vi "CoordLoadTemp.vi"(11 "appended path":path) -> (3 "CoordTempOut":T1[](array[typedef]))   [LabVIEW 2015]
uses:
  <vilib>/vision/Image Controls.llb/IMAQ Image.ctl
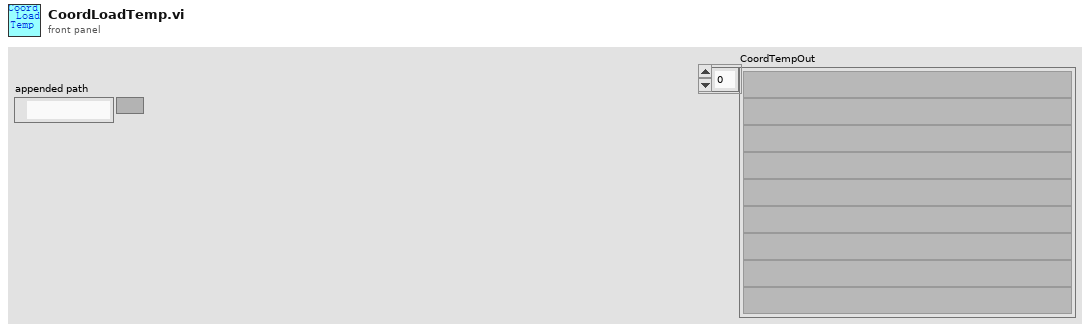
[diagram p1: front panel]
types:
  T1 = typedef "IMAQ Image.ctl" = refnum<image>
  T2 = typedef "Image Type" = u32
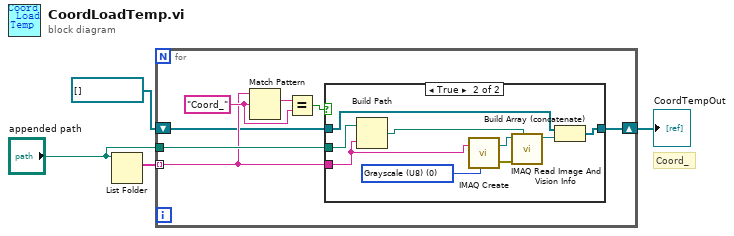
[diagram p0: block diagram]
diagram:
  # "Coord_"
  n1 = List Folder(path="appended path") -> (filenames=w4:string[])  [unwired: 3 in, 3 out]
  n2 = for {
    tunnel: w4 -> [w8] mode=indexing
    tunnel: "appended path" -> [w9]
    shift-right: [w5] -> w1
    shift-left: T1[] [] -> [w6]
    w10 = "Coord_" ("regular expression")
    n3 = Match Pattern(string=w8, regular expression=w10) -> (match substring=w11:string)  [unwired: 1 in, 3 out]
    n4 = Equal?(x=w11, y=w10) -> (x = y?=w7:bool)
    n5 = case shown="True" w7 {
      tunnel: w9 -> [_ w21]
      tunnel: w8 -> [_ w17]
      tunnel: [w12 w15] -> w5
      tunnel: w6 -> [w12 w14]
      frame False {
      }
      frame True {
        w20 = T2 0 items=["Grayscale (U8)", "Grayscale (I16)", "Grayscale (SGL)", "Complex (CSG)", "RGB (U32)", "HSL (U32)", "RGB (U64)", "Grayscale (U16)"] ("Image Type")
        n6 = Build Path(base path=w21, name or relative path=w17) -> (appended path=w18:path)
        n7 = call "IMAQ Create"("Image Name"=w17, "Image Type"=w20) -> ("New Image"=w19:T1, "error out"=w13:errorcluster)  [unwired: 3 in]
        n8 = call "IMAQ Read Image And Vision Info"("File Path"=w18, "error in (no error)"=w13, "Image"=w19) -> ("Image Out"=w16:T1)  [unwired: 6 in, 2 out]
        n9 = Build Array (concatenate)(w14, w16) -> (w15:T1[])
      }
    }
  }
  "CoordTempOut" <- w1
